vi "Init from Alternating Colors.vi"(8 "error in":errorcluster, 9 "Color Not Equal":T1=enum."AntiqueWhite", 10 "Color Equal":T1) -> (0 "error out":errorcluster, 3 "Cell View Alternating Back Color out":refnum<class "Cell View Alternating Back Color.lvclass">)   [LabVIEW 2023, in "SourceGrid.lvlib" / "Cell View Alternating Back Color.lvclass"]
uses:
  Cell View Alternating Back Color.lvclass
  Cell View/Cell View.lvclass
  Cell View Alternating Back Color.lvclass/Cell View Alternating Back Color.ctl
  System.Drawing.Color.ctl
  SourceGrid.lvlib
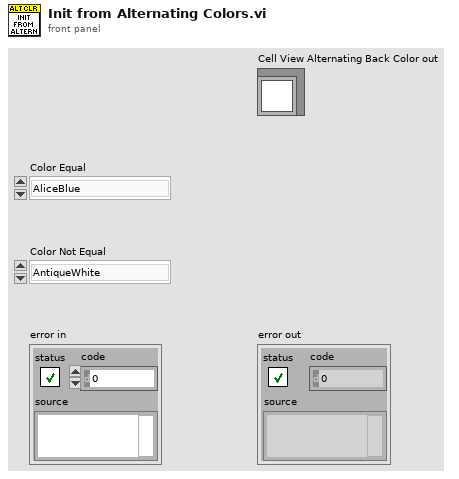
[diagram p1: front panel]
types:
  T1 = typedef "SourceGrid.lvlib/System.Drawing.Color.ctl" = enum16{"AliceBlue", "AntiqueWhite", "Aqua", "Aquamarine", "Azure", "Beige", "Bisque", "Black", "BlanchedAlmond", "Blue", "BlueViolet", "Brown", "BurlyWood", "CadetBlue", "Chartreuse", "Chocolate", "Coral", "CornflowerBlue", "Cornsilk", "Crimson", "Cyan", "DarkBlue", "DarkCyan", "DarkGoldenrod", "DarkGray", "DarkGreen", "DarkKhaki", "DarkMagenta", "DarkOliveGreen", "DarkOrange", "DarkOrchid", "DarkRed", "DarkSalmon", "DarkSeaGreen", "DarkSlateBlue", "DarkSlateGray", "DarkTurquoise", "DarkViolet", "DeepPink", "DeepSkyBlue", "DimGray", "DodgerBlue", "Firebrick", "FloralWhite", "ForestGreen", "Fuchsia", "Gainsboro", "GhostWhite", "Gold", "Goldenrod", "Gray", "Green", "GreenYellow", "Honeydew", "HotPink", "IndianRed", "Indigo", "Ivory", "Khaki", "Lavender", "LavenderBlush", "LawnGreen", "LemonChiffon", "LightBlue", "LightCoral", "LightCyan", "LightGoldenrodYellow", "LightGray", "LightGreen", "LightPink", "LightSalmon", "LightSeaGreen", "LightSkyBlue", "LightSlateGray", "LightSteelBlue", "LightYellow", "Lime", "LimeGreen", "Linen", "Magenta", "Maroon", "MediumAquamarine", "MediumBlue", "MediumOrchid", "MediumPurple", "MediumSeaGreen", "MediumSlateBlue", "MediumSpringGreen", "MediumTurquoise", "MediumVioletRed", "MidnightBlue", "MintCream", "MistyRose", "Moccasin", "NavajoWhite", "Navy", "OldLace", "Olive", "OliveDrab", "Orange", "OrangeRed", "Orchid", "PaleGoldenrod", "PaleGreen", "PaleTurquoise", "PaleVioletRed", "PapayaWhip", "PeachPuff", "Peru", "Pink", "Plum", "PowderBlue", "Purple", "Red", "RosyBrown", "RoyalBlue", "SaddleBrown", "Salmon", "SandyBrown", "SeaGreen", "SeaShell", "Sienna", "Silver", "SkyBlue", "SlateBlue", "SlateGray", "Snow", "SpringGreen", "SteelBlue", "Tan", "Teal", "Thistle", "Tomato", "Transparent", "Turquoise", "Violet", "Wheat", "White", "WhiteSmoke", "Yellow"}
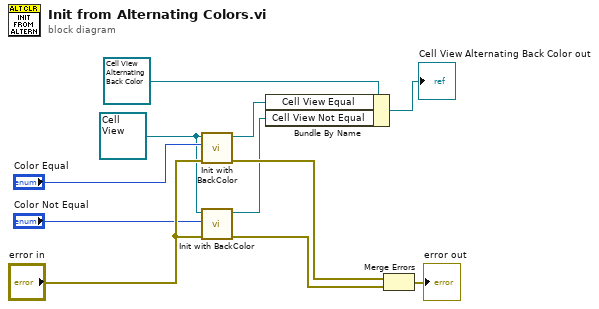
[diagram p0: block diagram]
diagram:
  w7 = refnum<class "Cell View.lvclass"> refnum ("Cell View in")
  n1 = call-dynamic "Init with BackColor.vi"("error in"="error in", "Color"="Color Equal", "Cell View in"=w7) -> ("error out"=w11:errorcluster, "Cell View out"=w3:refnum<class "Cell View.lvclass">)  [unwired: 7 in]
  n2 = call-dynamic "Init with BackColor.vi"("error in"="error in", "Color"="Color Not Equal", "Cell View in"=w7) -> ("error out"=w5:errorcluster, "Cell View out"=w2:refnum<class "Cell View.lvclass">)  [unwired: 7 in]
  n3 = Bundle By Name(cluster=refnum<class "Cell View Alternating Back Color.lvclass"> refnum ("Cell View Alternating Back Color in"), "Cell View Equal"=w3, "Cell View Not Equal"=w2) -> (→"Cell View Alternating Back Color out":refnum<class "Cell View Alternating Back Color.lvclass">)
  n4 = Merge Errors(w11, w5) -> (→"error out":errorcluster)
